vi "Test RegEx.vi"() -> ()   [LabVIEW 2014]
panel:
  out "offset past match":i32
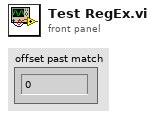
[diagram p1: front panel]
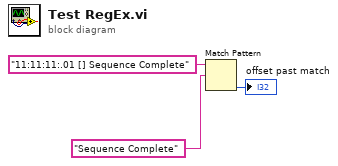
[diagram p0: block diagram]
diagram:
  n1 = Match Pattern(string="11:11:11:.01 [] Sequence Complete", regular expression="Sequence Complete" ("y")) -> (offset past match=→"offset past match":i32)  [unwired: 1 in, 3 out]
